vi "Controls.vi"() -> ()   [LabVIEW 2012]
panel:
  in  "Software Trigger":bool
  in  "Arm Acquisition Engine":bool
  out "Record Count":u32
  out "U256s Acquired":u32
  in  "DRAM Arbiter Config":T1={"write grant time (clocks)"=256, "read grant time (clocks)"=256}
  in  "DRAM FIFO Depth":u8(ring)=8 items=["4"=2, "8"=3, "16"=4, "32"=5, "64"=6, "128"=7, "256"=8, "512"=9, "1024"=10, "2048"=11, "4096"=12, "8192"=13, "16384"=14, "32768"=15, "65536"=16, "131072"=17, "262144"=18, "524288"=19, "1048576"=20, "2097152"=21, "4194304"=22, "8388608"=23, "16777216"=24, "33554432"=25, "67108864"=26, "134217728"=27, "268435456"=28, "536870912"=29, "1073741824"=30, "2147483648"=31, "4294967296"=32]
  in  "Record Parameters":T2={"Load Record Parameters?"=FALSE, "Pre Trigger Samples"=2, "Post Trigger Samples"=10, "Trigger Hold Off"=0, "Record Count"=1} {"Pre Trigger Samples" min=2}
  in  "Trigger Type":T3(ring)=enum."Software Trigger"
  out "U256s from DRAM FIFO":u32
  out "U256s to DRAM FIFO":u32
  out "Host FIFO Timed Out?":bool
  out "U64s to Host":u32
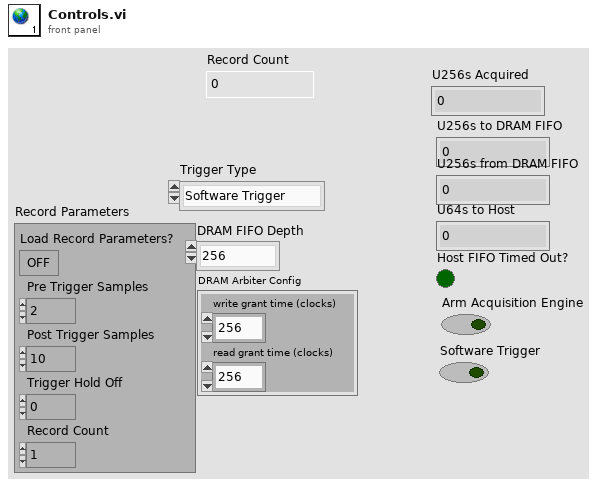
[diagram p1: front panel]
types:
  T1 = cluster{"write grant time (clocks)":u16, "read grant time (clocks)":u16}
  T2 = cluster{"Load Record Parameters?":bool, "Pre Trigger Samples":u32, "Post Trigger Samples":u32, "Trigger Hold Off":u32, "Record Count":u32}
  T3 = enum8{"Immediate Trigger", "Software Trigger", "External Digital Trigger", "Analog Trigger"}
diagram:
